vi "Send OVP.vi"(8 "error in (no error)":errorcluster, 11 "79XRP in":refnum<class "79XRP.lvclass">) -> (0 "error out":errorcluster, 3 "79XRP out":refnum<class "79XRP.lvclass">)   [LabVIEW 2019, in "79XRP.lvlib" / "79XRP.lvclass"]
uses:
  Library/79XRP.lvclass
  C:/Users/Public/Documents/Development/builds/Instruments/PowerSupply.lvlibp/Library/PowerSupply.lvclass
  Accessors/Read Local Resource.vi
  Accessors/Write Local Resource.vi
  <instrlib>/Keysight RP7900 Series/Keysight RP7900 Series.lvlib
  builds/Engine/Engine.lvlibp/Project/Engine.lvclass
  C:/Users/Public/Documents/Development/builds/Engine/Engine.lvlibp/Project/Engine.lvclass
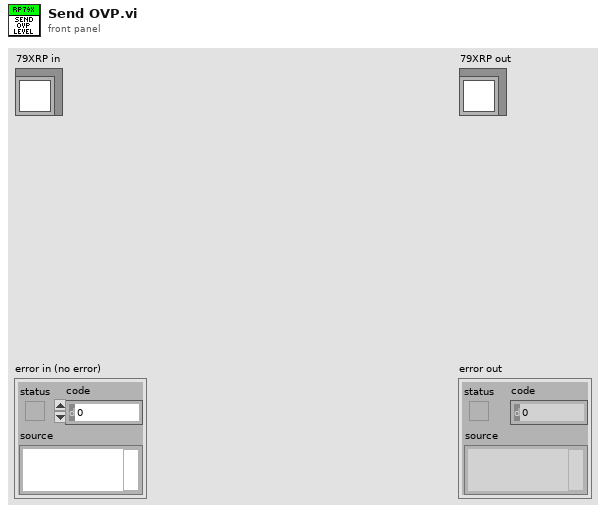
[diagram p1: front panel]
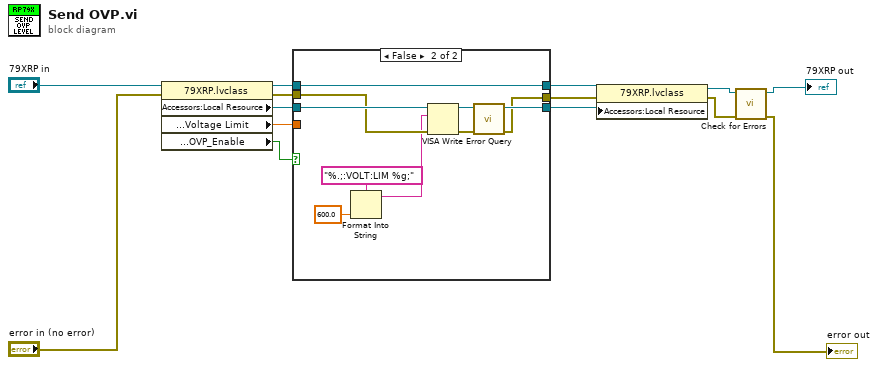
[diagram p0: block diagram]
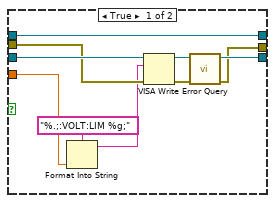
[diagram p2: hidden frame]
diagram:
  n1 = property class="79XRP.lvclass"(reference="79XRP in", error in="error in (no error)") -> (reference out=w6:refnum<class "79XRP.lvclass">, error out=w10:errorcluster, "Accessors:Local Resource"=w13:refnum<visa-resource-name>, "Accessors:Setting:Protection:Voltage Limit"=w11:dbl, "Accessors:Setting:Protection:OVP_Enable"=w7:bool)
  n2 = case shown="False" w7 {
    tunnel: w13 -> [w21 w31]
    tunnel: [w20 w30] -> w12
    tunnel: w11 -> [w19 _]
    tunnel: w10 -> [w18 w29]
    tunnel: [w16 w27] -> w9
    tunnel: [w15 w26] -> w5
    tunnel: w6 -> [w15 w26]
    frame True {
      n3 = Format Into String(format string="%.;:VOLT:LIM %g;", w19) -> (resulting string=w17:string)  [unwired: 2 in, 1 out]
      n4 = VISA Write(VISA resource name=w21, write buffer=w17, error in (no error)=w18) -> (VISA resource name out=w22:refnum<visa-resource-name>, error out=w23:errorcluster)  [unwired: 1 out]
      n5 = call <instrlib>:"Error Query.vi"("error in (no error)"=w23, "VISA resource name"=w22) -> ("error out"=w16:errorcluster, "VISA resource name out"=w20:refnum<visa-resource-name>)  [unwired: 6 in, 2 out]
    }
    frame False {
      n6 = Format Into String(format string="%.;:VOLT:LIM %g;", 600.0 ("input 1")) -> (resulting string=w28:string)  [unwired: 2 in, 1 out]
      n7 = VISA Write(VISA resource name=w31, write buffer=w28, error in (no error)=w29) -> (VISA resource name out=w32:refnum<visa-resource-name>, error out=w33:errorcluster)  [unwired: 1 out]
      n8 = call <instrlib>:"Error Query.vi"("error in (no error)"=w33, "VISA resource name"=w32) -> ("error out"=w27:errorcluster, "VISA resource name out"=w30:refnum<visa-resource-name>)  [unwired: 6 in, 2 out]
    }
  }
  n9 = property class="79XRP.lvclass"(reference=w5, error in=w9, "Accessors:Local Resource"=w12) -> (reference out=w4:refnum<class "79XRP.lvclass">, error out=w3:errorcluster)
  n10 = call "Check for Errors.vi"("error in"=w3, "Engine in"=w4) -> ("error out"=→"error out":errorcluster, "Engine out"=→"79XRP out":refnum<class "79XRP.lvclass">)  [unwired: 8 in]
